vi "Reserve cDAQ.vi"(8 "error in (no error)":errorcluster, 10 "Array in":string[](array[string]), 11 "Physical Channel":string) -> (0 "error out":errorcluster, 3 "Array out":string[](array[string]))   [LabVIEW 2015, in "DAQmx Module Runtime.lvclass"]
uses:
  DAQmx Module Runtime.lvclass
  <vilib>/regexp/Match Regular Expression.xnode
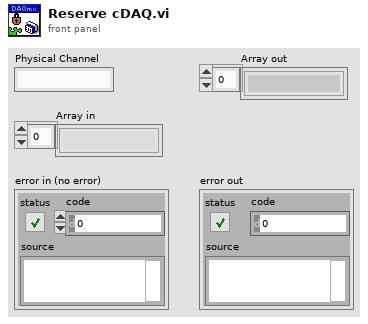
[diagram p1: front panel]
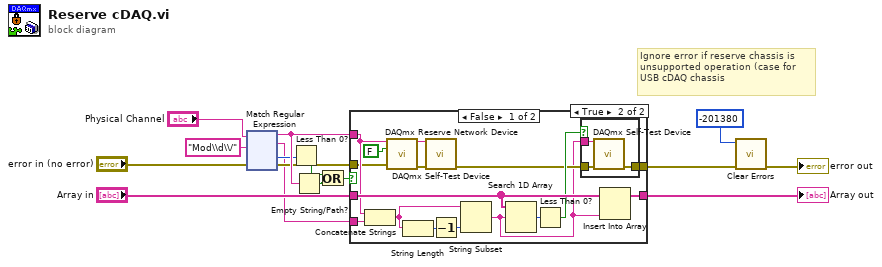
[diagram p0: block diagram]
diagram:
  # "Ignore error if reserve chassis is unsupported operation (case for USB cDAQ chassis"
  n1 = xnode "Match Regular Expression"("input string"="Physical Channel", "regular expression"="Mod\\d\\/", "error in"="error in (no error)") -> ("before match"=w12:string, "whole match"=w6:string, "offset past match"=w11:i32, "error out"=w8:errorcluster)  [unwired: 3 in, 1 out]
  n2 = Less Than 0?(x=w11) -> (x < 0?=w15:bool)
  n3 = Empty String/Path?(string/path=w12) -> (empty?=w14:bool)
  n4 = Or(x=w15, y=w14) -> (x .or. y?=w13:bool)
  n5 = case shown="False" w13 {
    tunnel: w6 -> [w31 _]
    tunnel: "Array in" -> [w29 w36]
    tunnel: w12 -> [w25 _]
    tunnel: w8 -> [w24 w37]
    tunnel: [w20 w36] -> w9
    tunnel: [w16 w37] -> w10
    frame False {
      n6 = Concatenate Strings(w25, w31) -> (w21:string)
      n7 = call <vilib>:"DAQmx Reserve Network Device.vi"("device in"=w25, "override reservation?"=FALSE, "error in"=w24) -> ("device out"=w27:tag, "error out"=w28:errorcluster)  [unwired: 11 in]
      n8 = String Length(string=w21) -> (length=w23:i32)
      n9 = call <vilib>:"DAQmx Self-Test Device.vi"("device in"=w27, "error in"=w28) -> ("error out"=w18:errorcluster)  [unwired: 13 in]
      n10 = Decrement(x=w23) -> (x-1=w22:i32)
      n11 = String Subset(string=w21, length (rest)=w22) -> (substring=w17:string)  [unwired: 1 in]
      n12 = Search 1D Array(1D array=w29, element=w17) -> (index of element=w30:i32)  [unwired: 1 in]
      n13 = Less Than 0?(x=w30) -> (x < 0?=w19:bool)
      n14 = case shown="True" w19 {
        tunnel: w18 -> [w32 w35]
        tunnel: w17 -> [_ w34]
        tunnel: [w32 w33] -> w16
        frame False {
        }
        frame True {
          n15 = call <vilib>:"DAQmx Self-Test Device.vi"("device in"=w34, "error in"=w35) -> ("error out"=w33:errorcluster)  [unwired: 13 in]
        }
      }
      n16 = Insert Into Array(array=w29, new element=w17) -> (w20:string[])  [unwired: 1 in]
    }
    frame True {
    }
  }
  "Array out" <- w9
  n17 = call <vilib>:"Clear Errors.vi"("error in (no error)"=w10, "specific error code to clear (0: all)"=-201380) -> ("error out"=→"error out":errorcluster)  [unwired: 4 in, 1 out]
